vi "PH_Sixpack_Switch.Action _Information.vi"(0 "i ref in":refnum<vi>, 5 "error IO":errorcluster) -> (14 "i ref out":refnum<vi>, 19 "error out":errorcluster)   [LabVIEW 2014, in "PH_Sixpack_Switch.lvlib"]
doc: "In this VI the action of the _Position Proc Case is done."
uses:
  PH_Sixpack_Switch.lvlib
  PH_Common/PH_Common.lvlib
  PH_AxisGUI_BaseClass/PH_AxisGUI_BaseClass.lvlib
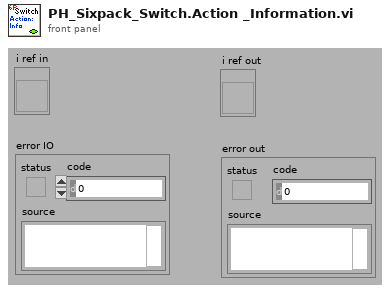
[diagram p1: front panel]
types:
  T1 = enum8{"Enabled", "Disabled", "Disabled and Grayed Out"}
  T2 = typedef "PH_AxisGUI_BaseClass.lvlib/PH_AxisGUI_BaseClass.i attribute.ctl" = cluster{"Axes":T3[]}
  T3 = typedef "PH_AxisGUI_BaseClass.lvlib/PH_AxisGUI_BaseClass.Axis Attributes.ctl" = cluster{"Axis GUI Refs":T4, "Address":T5, "Name":string, "Label \"Back\"":string, "Labell \"Forth\"":string, "Moving?":bool}
  T4 = typedef "PH_AxisGUI_BaseClass.lvlib/PH_AxisGUI_BaseClass.Axis GUI Refs.ctl" = cluster{"Back":refnum<vi>, "Forth":refnum<vi>, "Status":refnum<vi>, "Target":refnum<vi>, "Address":refnum<vi>, "Status Bar":refnum<vi>, "Settings":refnum<vi>, "Activity":refnum<vi>, "Clear Error":refnum<vi>}
  T5 = typedef "PH_Stepmotor_BaseClass.lvlib/PH_Stepmotor_BaseClass.Axis Address.ctl" = cluster{"Instance":string, "Motor Nr":i32}
  T6 = typedef "PH_Sixpack_Switch.lvlib/PH_Sixpack_Switch.i attribute.ctl" = cluster{"GUI Refs":cluster{"Delete":refnum<vi>, "Move":refnum<vi>, "Direction":refnum<vi>}, "remote controlled?":bool, "Move":bool, "Direction":T7}
  T7 = typedef "PH_Stepmotor_BaseClass.lvlib/PH_Stepmotor_BaseClass.Axis Direction.ctl" = enum16{"forward", "backward"}
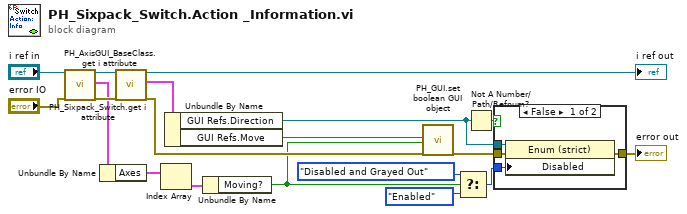
[diagram p0: block diagram]
diagram:
  n1 = call "PH_AxisGUI_BaseClass.get i attribute.vi"("i ref in"="i ref in", "error in (no error)"="error IO") -> ("i ref out"=w5:refnum<vi>, "i attribute"=w4:T2, "error out"=w7:errorcluster)  [unwired: 15 in]
  n2 = Unbundle By Name(w4) -> ("Axes"=w3:T3[])
  n3 = call "PH_Sixpack_Switch.get i attribute.vi"("i ref in"=w5, "error in (no error)"=w7) -> ("i ref out"=→"i ref out":refnum<vi>, "i attribute"=w17:T6, "error out"=w9:errorcluster)  [unwired: 15 in]
  n4 = Index Array(array=w3) -> (element=w2:T3)  [unwired: 1 in]
  n5 = Unbundle By Name(w17) -> ("GUI Refs.Direction"=w13:refnum<vi>, "GUI Refs.Move"=w10:refnum<vi>)
  n6 = Unbundle By Name(w2) -> ("Moving?"=w1:bool)
  n7 = call "PH_GUI.set boolean GUI object.vi"("Boolean Knob GUI Ref"=w10, "Value"=w1, "error in (no error)"=w9) -> ("error out"=w8:errorcluster)  [unwired: 16 in]
  n8 = Select(t=T1."Disabled and Grayed Out" ("Disabled"), s=w1, f=T1."Enabled" ("Disabled")) -> (s? t:f=w14:T1)
  n9 = Not A Number/Path/Refnum?(number/path/refnum=w13) -> (NaN/Path/Refnum?=w16:bool)
  n10 = case shown="False" w16 {
    tunnel: w13 -> [w23 _]
    tunnel: w14 -> [w22 _]
    tunnel: w8 -> [w21 w24]
    tunnel: [w20 w24] -> w15
    frame False {
      n11 = property class="Enum (strict)"(reference=w23, error in=w21, "Disabled"=w22) -> (error out=w20:errorcluster)  [unwired: 1 out]
    }
    frame True {
    }
  }
  "error out" <- w15
